vi "Initialize.vi"(6 "通道输入":string, 7 "原始采样率[Hz]":i32, 8 "error in (no error)":errorcluster caption="错误输入（无错误）", 9 "引用":T1, 10 "显示采样率[Hz]":i32, 11 "TPlot 输入":refnum<class "TPlot.lvclass">) -> (0 "error out":errorcluster caption="错误输出", 3 "TPlot 输出":refnum<class "TPlot.lvclass">)   [LabVIEW 2018, in "DataDisplay.lvlib" / "TPlot.lvclass"]
uses:
  TPlot.lvclass
  TPlotRef.ctl
  TypeDefine/DD_DataStream.ctl
  <vilib>/Utility/miscctls.llb/LVPointTypeDef.ctl
  TypeDefine/DD_Command.ctl
  TPlot.lvclass/TPlot.ctl
  SubVI/DD_Parameter.vi
  DataDisplay.lvlib
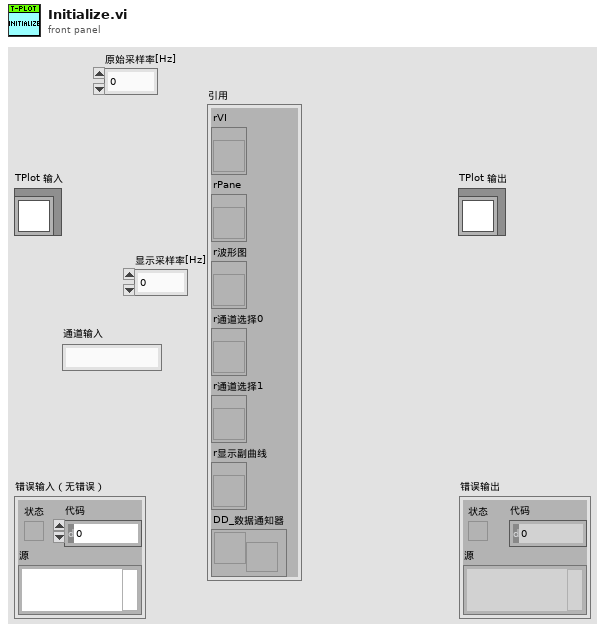
[diagram p1: front panel]
types:
  T1 = typedef "DataDisplay.lvlib/TPlot.lvclass/TPlotRef.ctl" = cluster{"rVI":refnum<vi>, "rPane":refnum<vi>, "r波形图":refnum<vi>, "r通道选择0":refnum<vi>, "r通道选择1":refnum<vi>, "r显示副曲线":refnum<vi>, "DD_数据通知器":refnum<notifier>}
  T2 = typedef "DataDisplay.lvlib/DD_Command.ctl" = cluster{"消息":string, "参数":variant}
  T3 = typedef "LVPointTypeDef.ctl" = cluster{"Horizontal":i16, "Vertical":i16}
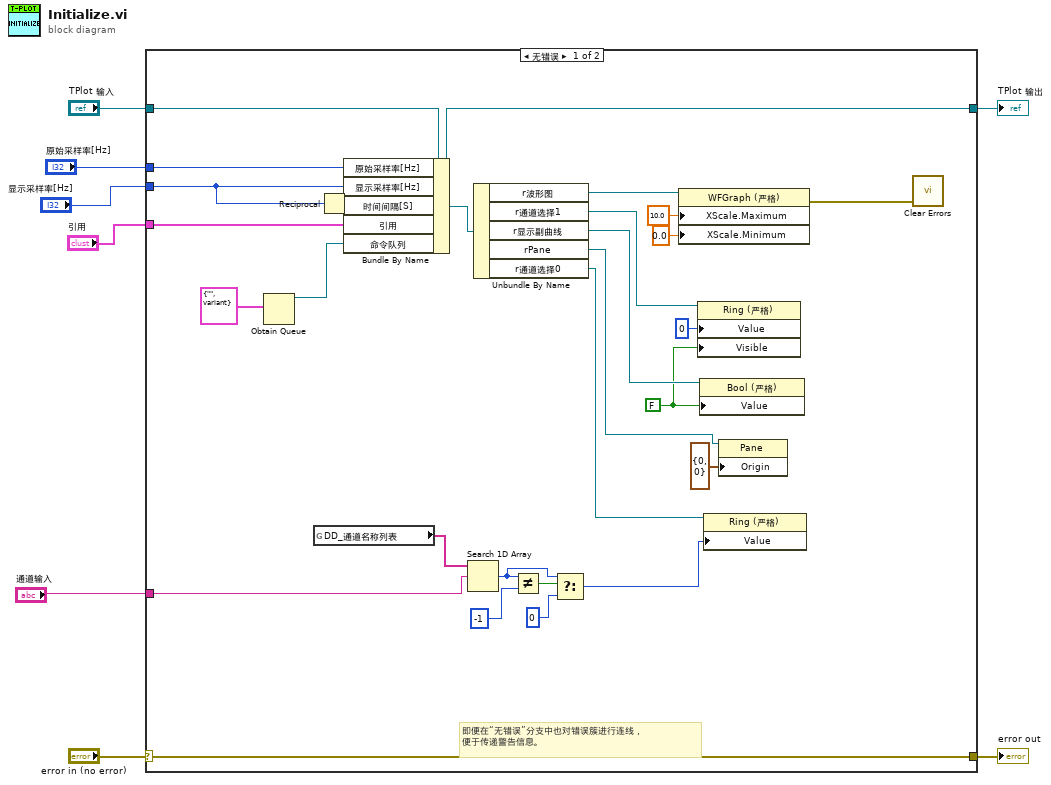
[diagram p0: block diagram]
diagram:
  n1 = case shown="无错误" "error in (no error)" {
    selector: "error in (no error)" -> [w34 w37]
    tunnel: [w34 w37] -> w7
    tunnel: [w33 w36] -> w5
    tunnel: "TPlot 输入" -> [w35 w36]
    tunnel: "显示采样率[Hz]" -> [w23 _]
    tunnel: "引用" -> [w20 _]
    tunnel: "原始采样率[Hz]" -> [w17 _]
    tunnel: "通道输入" -> [w11 _]
    frame No Error {
      w25 = FALSE ("值")
      # "即便在“无错误”分支中也对错误簇进行连线，\n便于传递警告信息。"
      n2 = Obtain Queue(element data type=T2 {"消息"="", "参数"=variant} ("簇")) -> (queue out=w19:refnum<queue>)  [unwired: 4 in, 2 out]
      n3 = global read "DD_Parameter.vi" "DD_通道名称列表"() -> (w16:string[])
      n4 = Reciprocal(x=w23) -> (1/x=w24:dbl)
      n5 = Bundle By Name(cluster=w35, "原始采样率[Hz]"=w17, "显示采样率[Hz]"=w23, "时间间隔[S]"=w24, "引用"=w20, "命令队列"=w19) -> (w33:refnum<class "TPlot.lvclass">)
      n6 = Search 1D Array(1D array=w16, element=w11) -> (index of element=w13:i32)  [unwired: 1 in]
      n7 = Unbundle By Name(w33) -> ("r波形图"=w32:refnum<vi>, "r通道选择1"=w26:refnum<vi>, "r显示副曲线"=w27:refnum<vi>, "rPane"=w22:refnum<vi>, "r通道选择0"=w10:refnum<vi>)
      n8 = Not Equal?(x=w13, y=-1) -> (x != y?=w14:bool)
      n9 = Select(t=w13, s=w14, f=0) -> (s? t:f=w9:i32)
      n10 = property class="WFGraph (严格)"(reference=w32, "XScale.Maximum"=10.0 ("X标尺.范围:最大值"), "XScale.Minimum"=0.0 ("X标尺.范围:最小值")) -> (error out=w29:errorcluster)  [unwired: 1 in, 1 out]
      n11 = property class="Ring (严格)"(reference=w26, "Value"=u16 0 ("值"), "Visible"=w25) -> ()  [unwired: 1 in, 2 out]
      n12 = property class="Bool (严格)"(reference=w27, "Value"=w25) -> ()  [unwired: 1 in, 2 out]
      n13 = property class="Ring (严格)"(reference=w10, "Value"=w9) -> ()  [unwired: 1 in, 2 out]
      n14 = property class="Pane"(reference=w22, "Origin"=T3 {"Horizontal"=0, "Vertical"=0} ("原点")) -> ()  [unwired: 1 in, 2 out]
      n15 = call <vilib>:"Clear Errors.vi"("error in (no error)"=w29) -> ()  [unwired: 5 in, 2 out]
    }
    frame Error {
    }
  }
  "error out" <- w7
  "TPlot 输出" <- w5
